vi "data_ID_impact_2.vi"(6 "Sensor Lookup Indices":i32[](array[numeric]), 7 "Start Z_Threshold":dbl format="%#_13g", 8 "error in (no error)":errorcluster, 9 "Pkt Size":i32, 10 "Gains":dbl[](array[numeric]), 11 "Byte Stream File in":refnum<file>) -> (0 "error out":errorcluster, 2 "Sensor_Tare":dbl[][](array[numeric]), 3 "Byte Stream File out":refnum<file>, 4 "N_end":i32, 5 "N_start":i32)   [LabVIEW 2018]
uses:
  <vilib>/Analysis/baseanly.llb/Mean (DBL).vi
  <vilib>/Analysis/NI_AALBase.lvlib
panel:
  out "Sensor Output - Position (mm)":dbl[][][](array[numeric])
  out "standard deviation":dbl format="%0.2f"
  out "mean":dbl format="%0.5f"
  out "Waveform Graph":dbl[](graph)
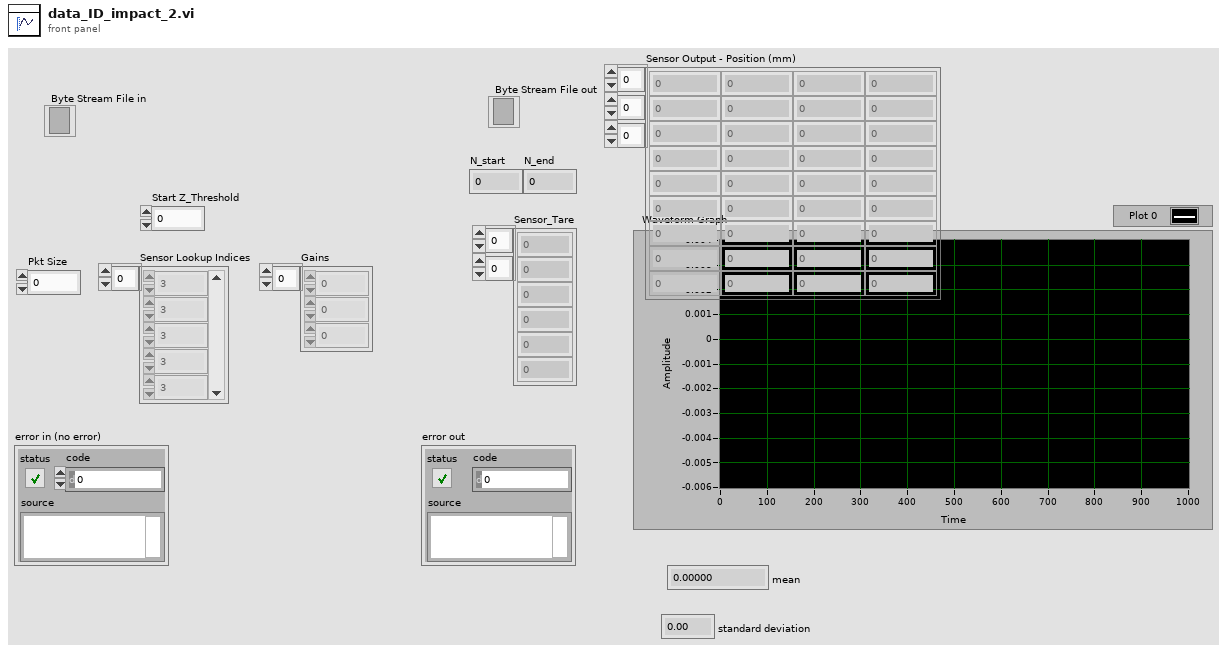
[diagram p1: front panel]
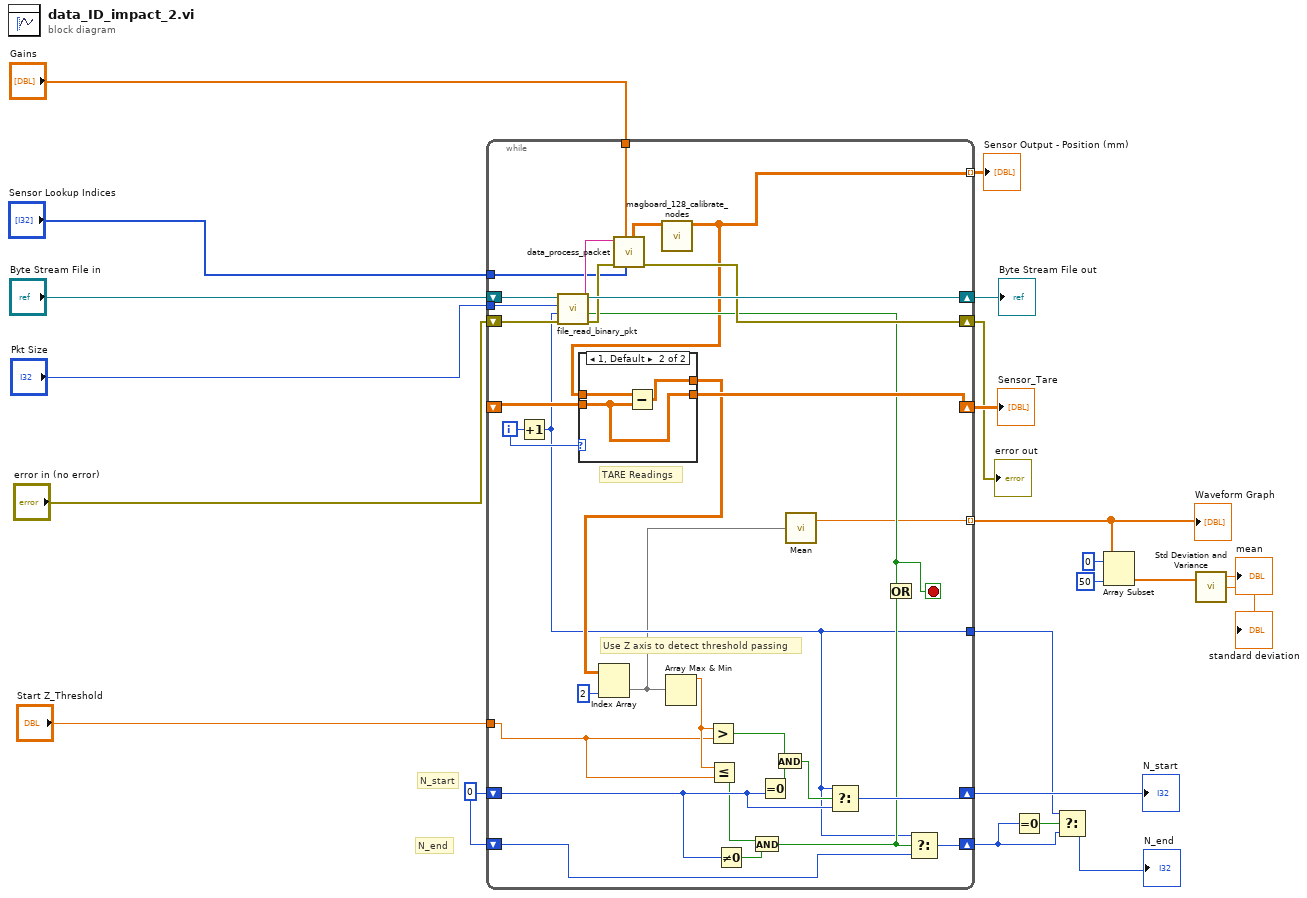
[diagram p0: block diagram]
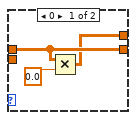
[diagram p2: hidden frame]
diagram:
  w15 = 0
  # "N_end"
  # "N_start"
  n1 = while {
    tunnel: "Pkt Size" -> [w53]
    shift-right: [w51] -> w18
    shift-left: "Byte Stream File in" -> [w54]
    shift-right: [w44] -> w20
    shift-left: "error in (no error)" -> [w50]
    shift-right: [w45] -> w22
    shift-left: _ -> [w46]
    tunnel: "Gains" -> [w43]
    shift-right: [w36] -> w14
    shift-left: w15 -> [w35]
    shift-right: [w32] -> w8
    shift-left: w15 -> [w31]
    tunnel: "Sensor Lookup Indices" -> [w29]
    tunnel: "Start Z_Threshold" -> [w28]
    tunnel: [w27] -> w9
    tunnel: [w24] -> w7 mode=indexing
    tunnel: [w23] -> w1 mode=indexing
    i -> [w52]
    stop <- w26 stop-if-true
    # "Use Z axis to detect threshold passing"
    # "TARE Readings"
    n2 = Increment(x=w52) -> (x+1=w27:i32)
    n3 = call "file_read_binary_pkt.vi"("error in (no error)"=w50, "Packet No."=w27, "Pkt Size(bytes)"=w53, "Byte Stream File in"=w54) -> ("error out"=w48:errorcluster, "EOF?"=w26:bool, "Packet"=w49:string, "Byte Stream File out"=w51:refnum<file>)  [unwired: 4 in]
    n4 = call "data_process_packet.vi"("Sensor Lookup Indices"=w29, "Gains"=w43, "error in (no error)"=w48, "Binary Input Data"=w49) -> ("error out"=w44:errorcluster, "Sensors (uT)"=w47:dbl[][])  [unwired: 3 in, 3 out]
    n5 = call "magboard_128_calibrate_nodes.vi"("Sensor Input (mT)"=w47) -> ("Sensor Output - Position (mm)"=w23:dbl[][])  [unwired: 10 in]
    n6 = case shown="1, Default" w52 {
      tunnel: w23 -> [w57 w58]
      tunnel: w46 -> [_ w59]
      tunnel: [w57 w59] -> w45
      tunnel: [w56 w60] -> w41
      frame 0 {
        n7 = Multiply(x=w57, y=0.0) -> (x*y=w56:dbl[][])
      }
      frame 1, Default {
        n8 = Subtract(x=w58, y=w59) -> (x-y=w60:dbl[][])
      }
    }
    n9 = Index Array(array=w41, index (col)=2 ("disabled index (col)")) -> (element=w25:dbl[])  [unwired: 1 in]
    n10 = Array Max & Min(array=w25) -> (max value=w40:dbl)  [unwired: 3 out]
    n11 = Greater?(x=w40, y=w28) -> (0:w39:bool)
    n12 = Less Or Equal?(x=w40, y=w28) -> (x <= y?=w33:bool)
    n13 = Not Equal To 0?(x=w35) -> (x != 0?=w34:bool)
    n14 = And(x=w33, y=w34) -> (x .and. y?=w30:bool)
    n15 = Equal To 0?(x=w35) -> (x = 0?=w38:bool)
    n16 = And(x=w39, y=w38) -> (x .and. y?=w37:bool)
    n17 = call-poly <vilib>:"Mean.vi"("X"=w25) -> ("mean"=w24:dbl)  [unwired: 1 out]
    n18 = Select(t=w27, s=w37, f=w35) -> (s? t:f=w36:i32)
    n19 = Or(x=w26, y=w30) -> ()  [unwired: 1 out]
    n20 = Select(t=w27, s=w30, f=w31) -> (s? t:f=w32:i32)
  }
  "Sensor_Tare" <- w22
  "error out" <- w20
  "Byte Stream File out" <- w18
  "N_start" <- w14
  "Waveform Graph" <- w7
  "Sensor Output - Position (mm)" <- w1
  n21 = Equal To 0?(x=w8) -> (x = 0?=w11:bool)
  n22 = Select(t=w9, s=w11, f=w8) -> (s? t:f=→"N_end":i32)
  n23 = Array Subset(array=w7, index=0, length=50) -> (w5:dbl[])
  n24 = call <vilib>:"Std Deviation and Variance.vi"("X"=w5) -> ("mean"=→"mean":dbl, "standard deviation"=→"standard deviation":dbl)  [unwired: 1 in, 1 out]
